vi "PropertyListAddAll.vi"(10 "VITag":string, 11 "PropertyList in":refnum<vi>) -> (3 "PropertyList out":refnum<vi>)   [LabVIEW 2021, in "VIPropertyPicker.lvlib"]
uses:
  VIPropertyPicker.lvlib
  f4f8af71-cf86-431e-bacc-fe96e0df66e8.vi
  <vilib>/Comparison/Equal/Equal Functor/Equal Functor.lvclass
  lib/SetGetControlValue/SetGetControlValue.lvlib
panel:
  in  "error in (no error)":errorcluster
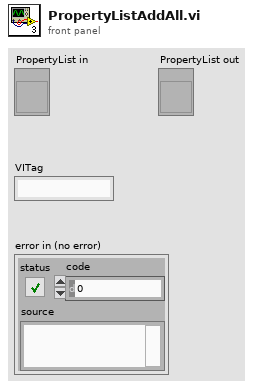
[diagram p1: front panel]
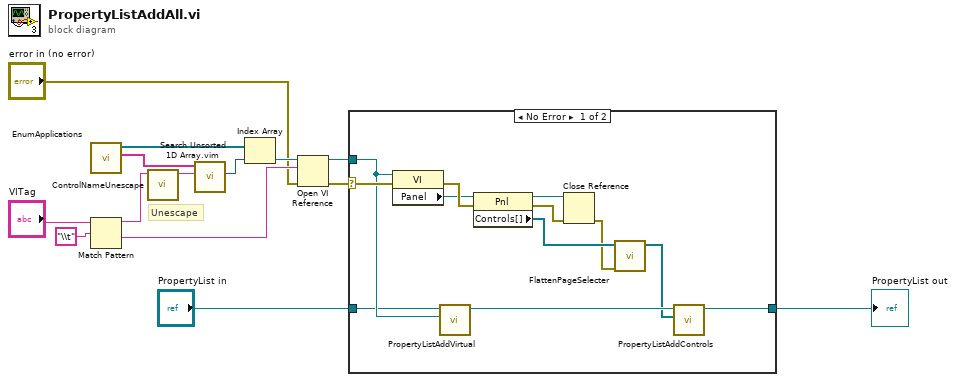
[diagram p0: block diagram]
diagram:
  # "Unescape"
  n1 = call "EnumApplications.vi"() -> ("Application Names"=w12:string[], "Application References"=w8:refnum<vi>[])  [unwired: 9 in, 1 out]
  n2 = Match Pattern(string="VITag", regular expression="\\t") -> (before substring=w11:string, after substring=w6:string)  [unwired: 1 in, 2 out]
  n3 = call "ControlNameUnescape.vi"("escaped string"=w11) -> ("label"=w10:string)  [unwired: 10 in]
  n4 = call "Search Unsorted 1D Array.vim"("element"=w10, "unsorted 1D array"=w12) -> ("index of element"=w9:i32)  [unwired: 9 in]
  n5 = Index Array(array=w8, index=w9) -> (element=w7:refnum<vi>)
  n6 = Open VI Reference(application reference (local)=w7, vi path=w6, error in (no error)="error in (no error)") -> (vi reference=w3:refnum<vi>, error out=w4:errorcluster)  [unwired: 3 in]
  n7 = case shown="No Error" w4 {
    selector: w4 -> [w23 _]
    tunnel: w3 -> [w22 _]
    tunnel: "PropertyList in" -> [w21 w27]
    tunnel: [w19 w27] -> w1
    frame No Error {
      n8 = property class="VI"(reference=w22, error in=w23) -> (error out=w25:errorcluster, "Panel"=w24:refnum<vi>)  [unwired: 1 out]
      n9 = call "PropertyListAddVirtual.vi"("vi reference"=w22, "Property List in"=w21) -> ("Property List out"=w20:refnum<vi>)  [unwired: 9 in]
      n10 = property class="Pnl"(reference=w24, error in=w25) -> (reference out=w17:refnum<vi>, error out=w16:errorcluster, "Controls[]"=w26:refnum<vi>[])
      n11 = Close Reference(reference=w17, error in (no error)=w16) -> (error out=w15:errorcluster)
      n12 = call "FlattenPageSelecter.vi"("error in (no error)"=w15, "Controls[]"=w26) -> ("Flatten[]"=w18:refnum<vi>[])  [unwired: 8 in, 1 out]
      n13 = call "PropertyListAddControls.vi"("Controls[]"=w18, "TreeControl in"=w20) -> ("TreeControl out"=w19:refnum<vi>)  [unwired: 9 in]
    }
    frame Error {
    }
  }
  "PropertyList out" <- w1
